vi "niRFSTS DCPower Configure Voltage Source.vi"(8 "error in":errorcluster, 9 "Voltage Source Setting per Pin":T1(array[cluster]) {"Sense" items=["Local"=1008, "Remote"=1009]}, 10 "Pins":string[](array[string])=["VCC"], 11 "Semiconductor Module Context":T2) -> (0 "error out":errorcluster)   [LabVIEW 2014]
uses:
  <vilib>/NI_TestStand_SemiconductorModule/NI_TestStand_Semiconductor_Module.lvlibp/PinMap/General/SemiconductorModuleContext.ctl
  <instrlib>/niDCPower/nidcpower.llb/niDCPower Output Function.ctl
  <instrlib>/niDCPower/nidcpower.llb/niDCPower Source Mode.ctl
  <vilib>/NI_TestStand_SemiconductorModule/NI_TestStand_Semiconductor_Module.lvlibp/PinMap/DC Power/PinToNIDCPowerSession.vi
  <vilib>/NI_TestStand_SemiconductorModule/NI_TestStand_Semiconductor_Module.lvlibp
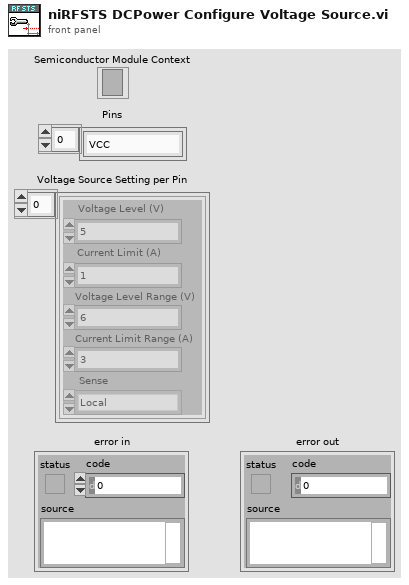
[diagram p1: front panel]
types:
  T1 = cluster{"Voltage Level (V)":dbl, "Current Limit (A)":dbl, "Voltage Level Range (V)":dbl, "Current Limit Range (A)":dbl, "Sense":i32}[]
  T2 = typedef "NI_TestStand_Semiconductor_Module.lvlibp/SemiconductorModuleContext.ctl" = refnum<k7>
  T3 = typedef "niDCPower Source Mode.ctl" = i32
  T4 = typedef "niDCPower Output Function.ctl" = i32
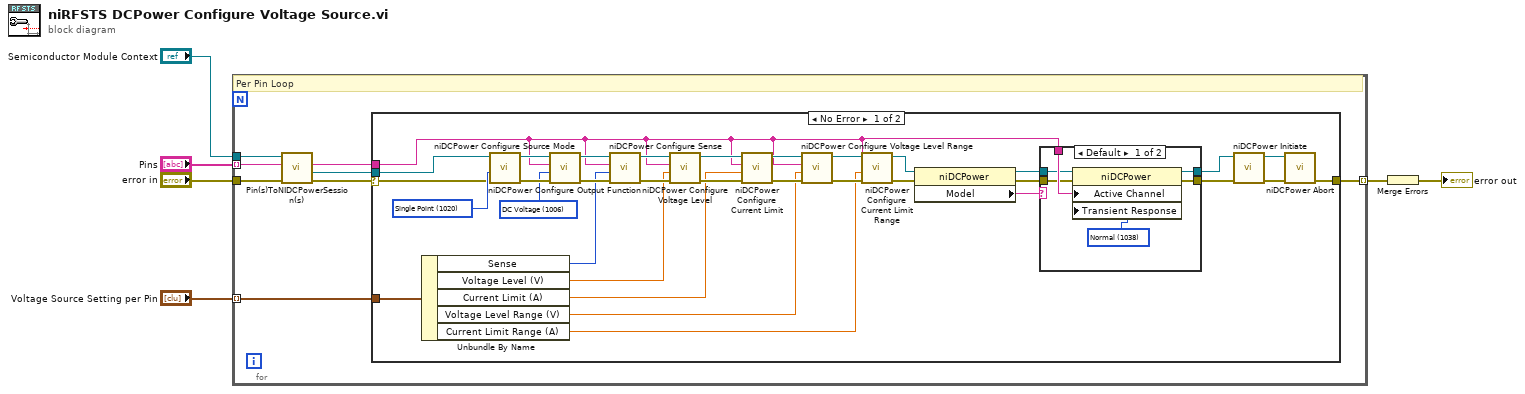
[diagram p0: block diagram]
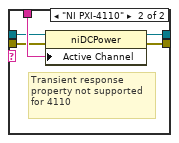
[diagram p2: hidden frame]
diagram:
  n1 = for {
    tunnel: "Semiconductor Module Context" -> [w12]
    tunnel: [w14] -> w3 mode=indexing
    tunnel: "Voltage Source Setting per Pin" -> [w13] mode=indexing
    tunnel: "Pins" -> [w10] mode=indexing
    tunnel: "error in" -> [w7]
    # "Per Pin Loop"
    n2 = call-poly <vilib>:"Pin(s)ToNIDCPowerSession(s).vi"("error in (no error)"=w7, "Pin"=w10, "Semiconductor Module Context"=w12) -> ("error out"=w8:errorcluster, "Instrument Session"=w11:refnum<k15>, "Channel List"=w9:string)  [unwired: 4 in, 2 out]
    n3 = case shown="No Error" w8 {
      selector: w8 -> [w16 w59]
      tunnel: [w18 w59] -> w14
      tunnel: w13 -> [w29 _]
      tunnel: w11 -> [w15 _]
      tunnel: w9 -> [w17 _]
      frame No Error {
        w43 = T3 1020 items=["Single Point"=1020, "Sequence"=1021] ("source mode")
        w32 = T4 1006 items=["DC Voltage"=1006, "DC Current"=1007] ("output function")
        n4 = Unbundle By Name(w29) -> ("Sense"=w28:i32, "Voltage Level (V)"=w27:dbl, "Current Limit (A)"=w26:dbl, "Voltage Level Range (V)"=w25:dbl, "Current Limit Range (A)"=w24:dbl)
        n5 = call <instrlib>:"niDCPower Configure Source Mode.vi"("error in (no error)"=w16, "source mode"=w43, "instrument handle"=w15) -> ("error out"=w35:errorcluster, "instrument handle out"=w36:refnum<k15>)  [unwired: 7 in]
        n6 = call <instrlib>:"niDCPower Configure Output Function.vi"("error in (no error)"=w35, "output function"=w32, "channel name"=w17, "instrument handle"=w36) -> ("error out"=w34:errorcluster, "instrument handle out"=w33:refnum<k15>)  [unwired: 6 in]
        n7 = call <instrlib>:"niDCPower Configure Sense.vi"("error in (no error)"=w34, "sense"=w28, "channel name"=w17, "instrument handle"=w33) -> ("error out"=w41:errorcluster, "instrument handle out"=w42:refnum<k15>)  [unwired: 6 in]
        n8 = call <instrlib>:"niDCPower Configure Voltage Level.vi"("error in (no error)"=w41, "voltage level"=w27, "channel name"=w17, "instrument handle"=w42) -> ("error out"=w31:errorcluster, "instrument handle out"=w30:refnum<k15>)  [unwired: 6 in]
        n9 = call <instrlib>:"niDCPower Configure Current Limit.vi"("error in (no error)"=w31, "current limit"=w26, "channel name"=w17, "instrument handle"=w30) -> ("error out"=w37:errorcluster, "instrument handle out"=w38:refnum<k15>)  [unwired: 6 in]
        n10 = call <instrlib>:"niDCPower Configure Voltage Level Range.vi"("error in (no error)"=w37, "voltage level range"=w25, "channel name"=w17, "instrument handle"=w38) -> ("error out"=w39:errorcluster, "instrument handle out"=w40:refnum<k15>)  [unwired: 6 in]
        n11 = call <instrlib>:"niDCPower Configure Current Limit Range.vi"("error in (no error)"=w39, "current limit range"=w24, "channel name"=w17, "instrument handle"=w40) -> ("error out"=w23:errorcluster, "instrument handle out"=w22:refnum<k15>)  [unwired: 6 in]
        n12 = property class="niDCPower"(reference=w22, error in=w23) -> (reference out=w20:refnum<k15>, error out=w21:errorcluster, "Model"=w19:string)
        n13 = case shown="Default" w19 {
          tunnel: [w53 w58] -> w45
          tunnel: [w52 w57] -> w44
          tunnel: w17 -> [w50 w56]
          tunnel: w21 -> [w49 w55]
          tunnel: w20 -> [w48 w54]
          frame Default {
            w51 = 1038 items=["Slow"=1041, "Normal"=1038, "Fast"=1039, "Custom"=1042] ("Source:Transient Response")
            n14 = property class="niDCPower"(reference=w48, error in=w49, "Active Channel"=w50, "Transient Response"=w51) -> (reference out=w52:refnum<k15>, error out=w53:errorcluster)
          }
          frame "NI PXI-4110" {
            # "Transient response\nproperty not supported\nfor 4110"
            n15 = property class="niDCPower"(reference=w54, error in=w55, "Active Channel"=w56) -> (reference out=w57:refnum<k15>, error out=w58:errorcluster)
          }
        }
        n16 = call <instrlib>:"niDCPower Initiate.vi"("error in (no error)"=w45, "instrument handle"=w44) -> ("error out"=w46:errorcluster, "instrument handle out"=w47:refnum<k15>)  [unwired: 8 in]
        n17 = call <instrlib>:"niDCPower Abort.vi"("error in (no error)"=w46, "instrument handle"=w47) -> ("error out"=w18:errorcluster)  [unwired: 8 in, 1 out]
      }
      frame Error {
      }
    }
  }
  n18 = Merge Errors(w3) -> (→"error out":errorcluster)
